vi "05 - Demonstration - High Throughput Transport Mechanism.vi"() -> ()   [LabVIEW 2012]
uses:
  <vilib>/picture/picture.llb/imagedata.ctl
panel:
  out "Events/sec":dbl caption="Events Throughput" format="%_4f events/sec"
  out "Picture 2":picture
  out "Picture 1":picture
  out "MB/sec":dbl caption="Data Throughput" format="%.2f MB/sec"
  out "Color Box 2":u32(colorbox)
  out "Color Box 1":u32(colorbox)
  # "Yo, so I heard User Events are 'kinda slow'\nGenerally, User Events are indeed not as performant as queues,\nyet they are unlikely to be a performance bottleneck in your application."
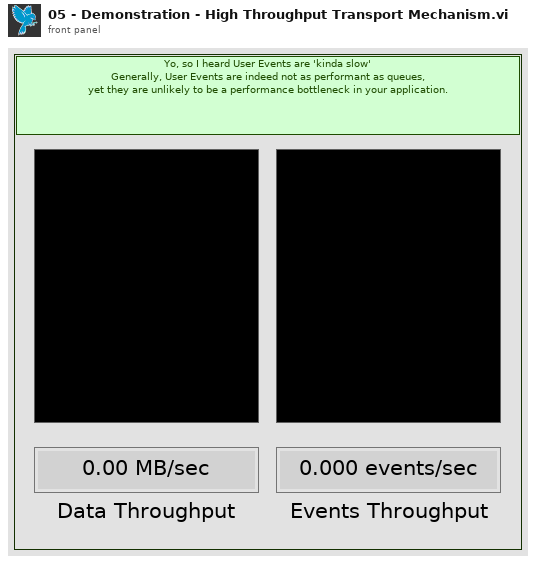
[diagram p1: front panel]
types:
  T1 = typedef "imagedata.ctl" = cluster{"image type":i32, "image depth":i32, "image":u8[], "mask":u8[], "colors":u32[], "Rectangle":cluster{"left":i16, "top":i16, "right":i16, "bottom":i16}}
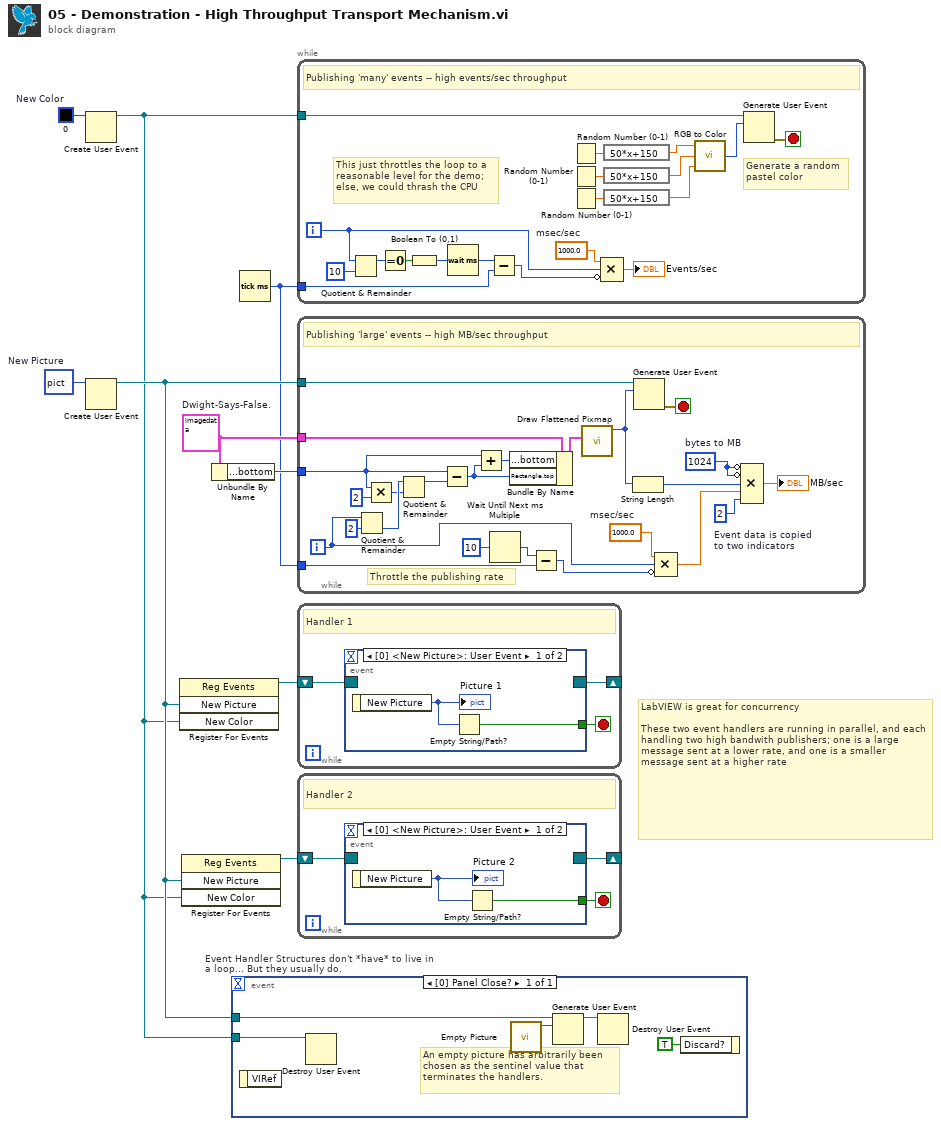
[diagram p0: block diagram]
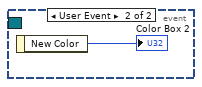
[diagram p2: hidden frame]
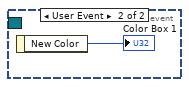
[diagram p3: hidden frame]
diagram:
  w4 = u32 0  # New Color
  w6 = T1 {"image type"=0, "image depth"=32, "image"=array[234768 elements], "mask"=array[7504 elements], "colors"=[], "Rectangle"={"left"=0, "top"=0, "right"=219, "bottom"=268}}  # Dwight-Says-False.
  w7 = picture data[5B]  # New Picture
  # "LabVIEW is great for concurrency\n\nThese two event handlers are running in parallel, and each handling two high bandwith publishers; one is a large message sent at a lower rate, and one is a smaller message sent at a higher rate"
  n1 = Create User Event(user event datatype=w4) -> (user event=w2:refnum<user-event>)  [unwired: 1 in, 1 out]
  n2 = Create User Event(user event datatype=w7) -> (user event=w3:refnum<user-event>)  [unwired: 1 in, 1 out]
  n3 = register-events(w3, w2) -> (reference out=w9:refnum<event-registration>)  [unwired: 2 in, 1 out]
  n4 = register-events(w3, w2) -> (reference out=w8:refnum<event-registration>)  [unwired: 2 in, 1 out]
  n5 = Unbundle By Name(w6) -> ("Rectangle.bottom"=w5:i16)
  n6 = event "Event Handler Structures don't *have* to live in a loop... But they usually do." shown="[0] Panel Close?" {
    selector: _ -> [_]
    dyn-events: _ -> [_]
    timeout: _ -> [_]
    tunnel: w3 -> [w12]
    tunnel: w2 -> [w14]
    event Panel Close? {
      # "An empty picture has arbitrarily been\nchosen as the sentinel value that\nterminates the handlers."
      n7 = event-data() -> ()  [unwired: 1 in, 1 out]
      n8 = Destroy User Event(user event=w14) -> ()  [unwired: 1 in, 1 out]
      n9 = call "Empty Picture"() -> ("empty picture"=w10:picture)
      n10 = Generate User Event(user event=w12, event data cluster=w10) -> (user event out=w11:refnum<user-event>)  [unwired: 1 in, 1 out]
      n11 = Destroy User Event(user event=w11) -> ()  [unwired: 1 in, 1 out]
      n12 = event-data("Discard?"=TRUE) -> ()  [unwired: 1 in, 1 out]
    }
  }
  n13 = Tick Count (ms)() -> (millisecond timer value=w1:u32)
  n14 = while {
    tunnel: w2 -> [w33]
    tunnel: w1 -> [w26]
    i -> [w15]
    stop <- w31 stop-if-true
    w25 = 1000.0  # msec/sec
    # "This just throttles the loop to a\nreasonable level for the demo;\nelse, we could thrash the CPU"
    # "Generate a random\npastel color"
    # "Publishing 'many' events -- high events/sec throughput"
    n15 = Quotient & Remainder(x=w15, y=10) -> (x-y*floor(x/y)=w29:i32)  [unwired: 1 out]
    n16 = Equal To 0?(x=w29) -> (x = 0?=w28:bool)
    n17 = Boolean To (0,1)(Boolean=w28) -> (0, 1=w22:i16)
    n18 = Wait (ms)(milliseconds to wait=w22) -> (millisecond timer value=w27:u32)
    n19 = Subtract(x=w27, y=w26) -> (x-y=w24:u32)
    n20 = Random Number (0-1)() -> (number: 0 to 1=w21:dbl)
    n21 = Random Number (0-1)() -> (number: 0 to 1=w19:dbl)
    n22 = Random Number (0-1)() -> (number: 0 to 1=w18:dbl)
    n23 = Compound Arithmetic op=MULTIPLY(w25, w15, invert w24) -> (→"Events/sec":dbl)
    n24 = expression code="50*x+150"(w21) -> (w20:dbl)
    n25 = expression code="50*x+150"(w19) -> (w16:dbl)
    n26 = expression code="50*x+150"(w18) -> (w17:dbl)
    n27 = call <vilib>:"RGB to Color.vi"("B"=w17, "G"=w16, "R"=w20) -> ("Color"=w32:u32)
    n28 = Generate User Event(user event=w33, event data cluster=w32) -> (error out=w31:errorcluster)  [unwired: 1 in, 1 out]
  }
  n29 = while {
    tunnel: w3 -> [w56]
    tunnel: w1 -> [w55]
    tunnel: w6 -> [w46]
    tunnel: w5 -> [w36]
    i -> [w34]
    stop <- w41 stop-if-true
    w35 = 2  # Event data is copied to two indicators
    w49 = 1024  # bytes to MB
    w53 = 1000.0  # msec/sec
    # "Throttle the publishing rate"
    # "Publishing 'large' events -- high MB/sec throughput"
    n30 = Quotient & Remainder(x=w34, y=2) -> (floor(x/y)=w45:i32)  [unwired: 1 out]
    n31 = Multiply(x=w36, y=i16 2) -> (x*y=w37:i16)
    n32 = Quotient & Remainder(x=w45, y=w37) -> (x-y*floor(x/y)=w40:i32)  [unwired: 1 out]
    n33 = Subtract(x=w36, y=w40) -> (x-y=w39:i32)
    n34 = Add(x=w36, y=w39) -> (x+y=w42:i32)
    n35 = Wait Until Next ms Multiple(millisecond multiple=u32 10 ("milliseconds to wait")) -> (millisecond timer value=w43:u32)
    n36 = Bundle By Name(cluster=w46, "Rectangle.bottom"=w42, "Rectangle.top"=w39) -> (w47:T1)
    n37 = Subtract(x=w43, y=w55) -> (x-y=w54:u32)
    n38 = call <vilib>:"Draw Flattened Pixmap.vi"("image data"=w47) -> ("new picture"=w48:picture)  [unwired: 8 in]
    n39 = String Length(string=w48) -> (length=w52:i32)
    n40 = Generate User Event(user event=w56, event data cluster=w48) -> (error out=w41:errorcluster)  [unwired: 1 in, 1 out]
    n41 = Compound Arithmetic op=MULTIPLY(w53, w34, invert w54) -> (w51:dbl)
    n42 = Compound Arithmetic op=MULTIPLY(invert w49, invert w49, w52, w51, w35) -> (→"MB/sec":dbl)
  }
  n43 = while {
    shift-right: [w59] -> _
    shift-left: w9 -> [w60]
    stop <- w58 stop-if-true
    # "Handler 1"
    n44 = event shown="[0] <New Picture>: User Event" {
      selector: w60 -> [_ _]
      dyn-events: [_ _] -> w59
      timeout: _ -> [_ _]
      tunnel: [w61 _] -> w58
      event User Event {
        n45 = event-data() -> ("New Picture"=w62:picture)  [unwired: 1 in]
        "Picture 1" <- w62
        n46 = Empty String/Path?(string/path=w62) -> (empty?=w61:bool)
      }
      event User Event {
        n47 = event-data() -> ("New Color"=→"Color Box 1":u32)  [unwired: 1 in]
      }
    }
  }
  n48 = while {
    shift-right: [w65] -> _
    shift-left: w8 -> [w66]
    stop <- w64 stop-if-true
    # "Handler 2"
    n49 = event shown="[0] <New Picture>: User Event" {
      selector: w66 -> [_ _]
      dyn-events: [_ _] -> w65
      timeout: _ -> [_ _]
      tunnel: [w67 _] -> w64
      event User Event {
        n50 = event-data() -> ("New Picture"=w68:picture)  [unwired: 1 in]
        "Picture 2" <- w68
        n51 = Empty String/Path?(string/path=w68) -> (empty?=w67:bool)
      }
      event User Event {
        n52 = event-data() -> ("New Color"=→"Color Box 2":u32)  [unwired: 1 in]
      }
    }
  }
